vi "Anode Purge Logic.vi"(10 "Purge Strategy":T1={"Strategy"=enum."FORCE OFF", "Purge Interval [s]"=30.0, "Purge Duration [s]"=1.0}, 11 "Purge State in":T4) -> (1 "Valve State":enum16{"CLOSED", "OPEN"}(ring), 3 "Purge State out":T4)   [LabVIEW 2024, in "Anode.lvlib"]
doc: "<b>Note:</b> This VI was modified by the <b>Validate DQMH Module</b> tool to turn off automatic error handling."
uses:
  Anode.lvlib
  Purge Valve State--cluster.ctl
  Purge Strategy--cluster.ctl
  Purge Strategy--enum.ctl
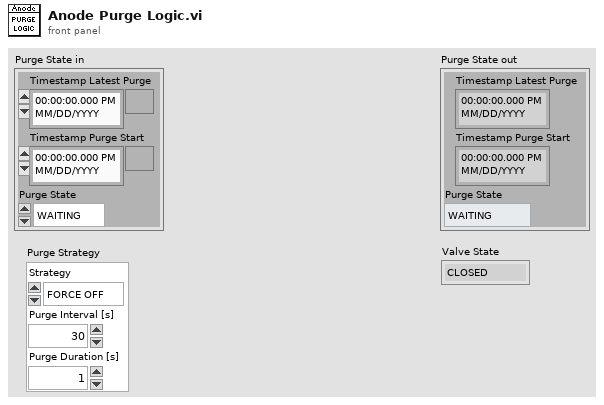
[diagram p1: front panel]
types:
  T1 = typedef "Anode.lvlib/Purge Strategy--cluster.ctl" = cluster{"Strategy":T2, "Purge Interval [s]":dbl, "Purge Duration [s]":dbl}
  T2 = typedef "Anode.lvlib/Purge Strategy--enum.ctl" = enum16{"FORCE OFF", "FORCE ON", "TIMED"}
  T3 = typedef "Anode.lvlib/Purge Valve State--cluster.ctl" = enum16{"WAITING", "PURGING"}
  T4 = cluster{"Timestamp Latest Purge":timestamp, "Timestamp Purge Start":timestamp, "Purge State":T3}
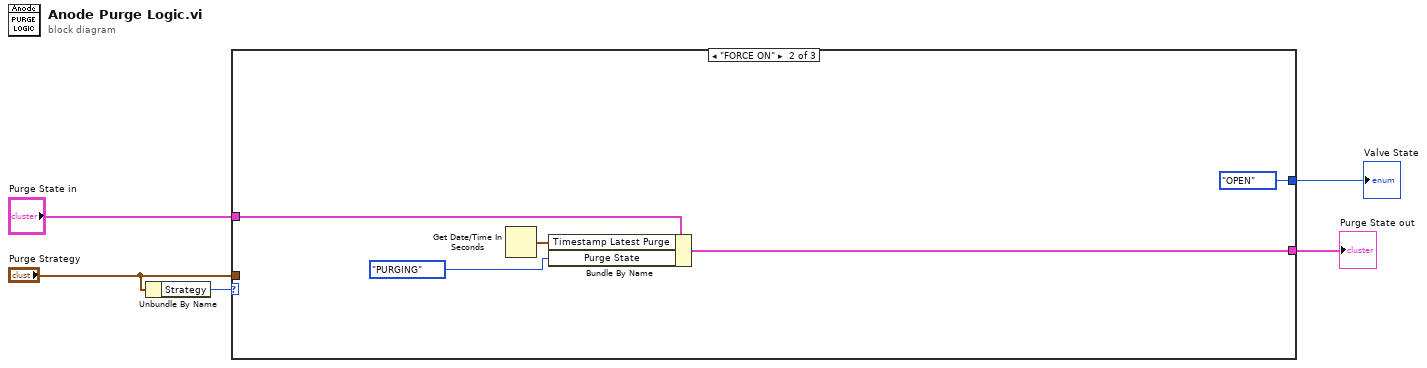
[diagram p0: block diagram]
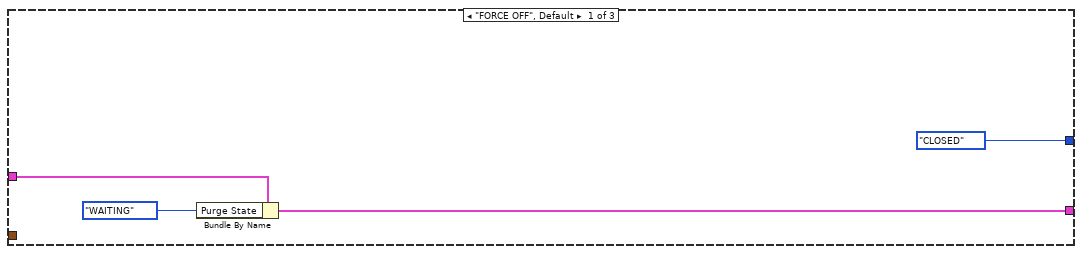
[diagram p2: hidden frame]
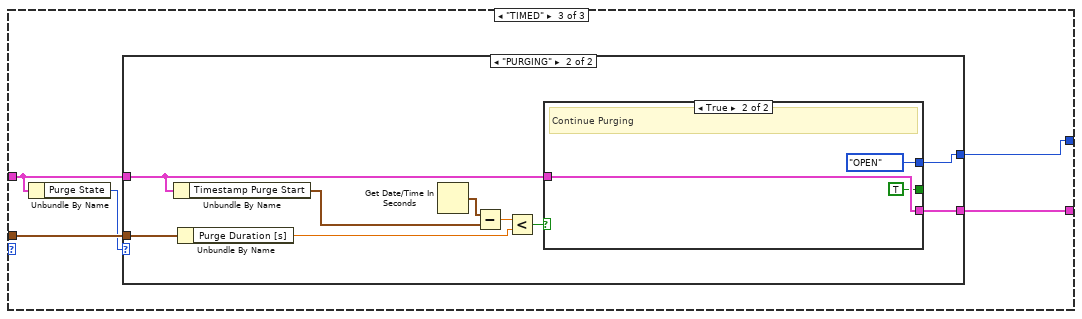
[diagram p3: hidden frame]
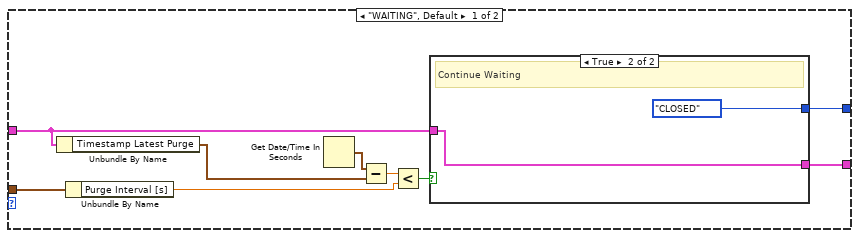
[diagram p4: hidden frame]
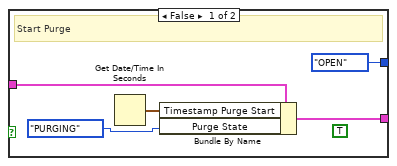
[diagram p5: hidden frame]
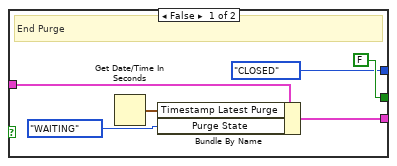
[diagram p6: hidden frame]
diagram:
  n1 = Unbundle By Name("Purge Strategy") -> ("Strategy"=w3:T2)
  n2 = case shown="\"FORCE ON\"" w3 {
    tunnel: "Purge Strategy" -> [_ _ w19]
    tunnel: [w7 w11 w18] -> w4
    tunnel: "Purge State in" -> [w8 w14 w16]
    tunnel: [enum16{"CLOSED", "OPEN"}."CLOSED" ("Valve State") enum16{"CLOSED", "OPEN"}."OPEN" ("Valve State") w15] -> w1
    frame "FORCE OFF", Default {
      n3 = Bundle By Name(cluster=w8, "Purge State"=Purge_Valve_State--cluster."WAITING") -> (w7:T4)
    }
    frame "FORCE ON" {
      n4 = Get Date/Time In Seconds() -> (seconds since 1Jan1904=w13:timestamp)
      n5 = Bundle By Name(cluster=w14, "Timestamp Latest Purge"=w13, "Purge State"=Purge_Valve_State--cluster."PURGING") -> (w11:T4)
    }
    frame "TIMED" {
      n6 = Unbundle By Name(w16) -> ("Purge State"=w17:T3)
      n7 = case shown="\"PURGING\"" w17 {
        tunnel: w19 -> [w24 w42]
        tunnel: [w21 w40] -> w18
        tunnel: w16 -> [w22 w38]
        tunnel: [w20 w36] -> w15
        frame "WAITING", Default {
          n8 = Unbundle By Name(w22) -> ("Timestamp Latest Purge"=w23:timestamp)
          n9 = Unbundle By Name(w24) -> ("Purge Interval [s]"=w26:dbl)
          n10 = Get Date/Time In Seconds() -> (seconds since 1Jan1904=w28:timestamp)
          n11 = Subtract(x=w28, y=w23) -> (x-y=w27:dbl)
          n12 = Less?(x=w27, y=w26) -> (x < y?=w25:bool)
          n13 = case shown="True" w25 {
            tunnel: [w32 w35] -> w21
            tunnel: w22 -> [w31 w35]
            tunnel: [enum16{"CLOSED", "OPEN"}."OPEN" ("Valve State") enum16{"CLOSED", "OPEN"}."CLOSED" ("Valve State")] -> w20
            frame False {
              (unwired) TRUE
              # "Start Purge"
              n14 = Get Date/Time In Seconds() -> (seconds since 1Jan1904=w33:timestamp)
              n15 = Bundle By Name(cluster=w31, "Timestamp Purge Start"=w33, "Purge State"=Purge_Valve_State--cluster."PURGING") -> (w32:T4)
            }
            frame True {
              # "Continue Waiting"
            }
          }
        }
        frame "PURGING" {
          n16 = Unbundle By Name(w38) -> ("Timestamp Purge Start"=w37:timestamp)
          n17 = Unbundle By Name(w42) -> ("Purge Duration [s]"=w41:dbl)
          n18 = Get Date/Time In Seconds() -> (seconds since 1Jan1904=w44:timestamp)
          n19 = Subtract(x=w44, y=w37) -> (x-y=w43:dbl)
          n20 = Less?(x=w43, y=w41) -> (x < y?=w39:bool)
          n21 = case shown="True" w39 {
            tunnel: [w47 w53] -> w40
            tunnel: w38 -> [w49 w53]
            tunnel: [FALSE TRUE] -> _
            tunnel: [enum16{"CLOSED", "OPEN"}."CLOSED" ("Valve State") enum16{"CLOSED", "OPEN"}."OPEN" ("Valve State")] -> w36
            frame False {
              # "End Purge"
              n22 = Get Date/Time In Seconds() -> (seconds since 1Jan1904=w48:timestamp)
              n23 = Bundle By Name(cluster=w49, "Timestamp Latest Purge"=w48, "Purge State"=Purge_Valve_State--cluster."WAITING") -> (w47:T4)
            }
            frame True {
              # "Continue Purging"
            }
          }
        }
      }
    }
  }
  "Purge State out" <- w4
  "Valve State" <- w1
